vi "Analog Trigger with Interleaving Select.vi"(0 "all channels":cluster{fxp<+/-,12,1>[]}[](array[cluster])=[{[0.0, 0.0, 0.0, 0.0, 0.0, 0.0, 0.0, 0.0, 0.0, 0.0, 0.0, 0.0, 0.0, 0.0, 0.0, 0.0]}, {[0.0, 0.0, 0.0, 0.0, 0.0, 0.0, 0.0, 0.0, 0.0, 0.0, 0.0, 0.0, 0.0, 0.0, 0.0, 0.0]}], 5 "config":T1, 7 "interleaving factor":u16) -> (4 "all channels delayed out":cluster{fxp<+/-,12,1>[]}[](array[cluster]), 6 "triggered":bool)   [LabVIEW 2018, in "GettingStarted_5785_FPGA.lvlib"]
uses:
  GettingStarted_5785_FPGA.lvlib
  1961724d-2c00-4db4-be5f-47e2776cd38e.vi
  db24aacc-3aa9-45e6-b75f-233848c1dcdd.vi
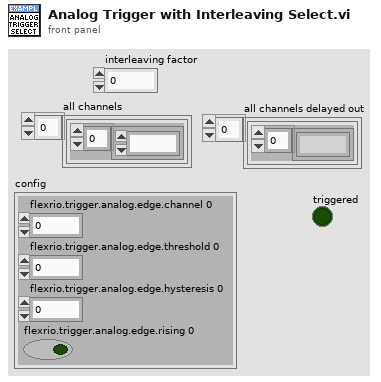
[diagram p1: front panel]
types:
  T1 = cluster{"flexrio.trigger.analog.edge.channel 0":fxp<+,2,2>, "flexrio.trigger.analog.edge.threshold 0":fxp<+/-,32,1>, "flexrio.trigger.analog.edge.hysteresis 0":fxp<+/-,32,1>, "flexrio.trigger.analog.edge.rising 0":bool}
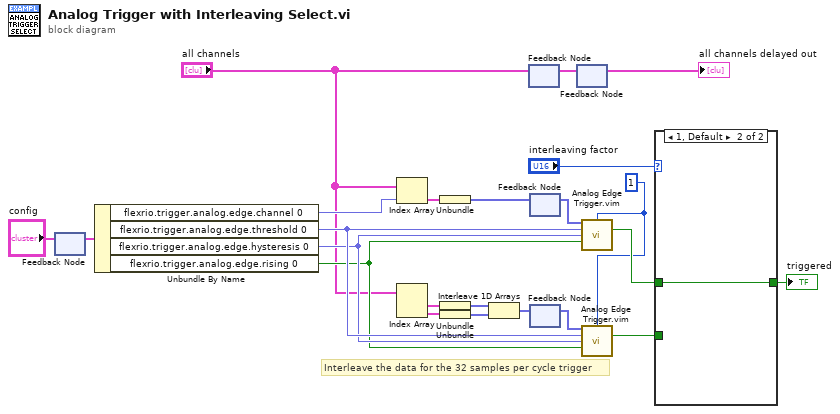
[diagram p0: block diagram]
diagram:
  w10 = u8 1 ("internal pipeline stages")
  # "Interleave the data for the 32 samples per cycle trigger"
  n1 = feedback #1() -> (w8:T1)  [unwired: 1 in]
  n2 = feedback-in #1("config") -> ()
  n3 = Unbundle By Name(w8) -> ("flexrio.trigger.analog.edge.channel 0"=w7:fxp<+,2,2>, "flexrio.trigger.analog.edge.threshold 0"=w6:fxp<+/-,32,1>, "flexrio.trigger.analog.edge.hysteresis 0"=w5:fxp<+/-,32,1>, "flexrio.trigger.analog.edge.rising 0"=w4:bool)
  n4 = Index Array(array="all channels", index=w7) -> (element=w16:cluster{fxp<+/-,12,1>[]})
  n5 = Index Array(array="all channels") -> (element #1=w19:cluster{fxp<+/-,12,1>[]}, element #2=w20:cluster{fxp<+/-,12,1>[]})  [unwired: 2 in]
  n6 = Unbundle(w16) -> (w17:fxp<+/-,12,1>[])
  n7 = Unbundle(w19) -> (w21:fxp<+/-,12,1>[])
  n8 = Unbundle(w20) -> (w22:fxp<+/-,12,1>[])
  n9 = Interleave 1D Arrays(w21, w22) -> (w23:fxp<+/-,12,1>[])
  n10 = feedback #2() -> (w2:cluster{fxp<+/-,12,1>[]}[])  [unwired: 1 in]
  n11 = feedback-in #2("all channels") -> ()
  n12 = feedback #3() -> (w15:fxp<+/-,12,1>[])  [unwired: 1 in]
  n13 = feedback-in #3(w17) -> ()
  n14 = feedback #4() -> (w18:fxp<+/-,12,1>[])  [unwired: 1 in]
  n15 = feedback-in #4(w23) -> ()
  n16 = feedback #5() -> (→"all channels delayed out":cluster{fxp<+/-,12,1>[]}[])  [unwired: 1 in]
  n17 = feedback-in #5(w2) -> ()
  n18 = call "Analog Edge Trigger.vim"("trigger channel data"=w15, "internal pipeline stages"=w10, "requested trigger level"=w6, "requested hysteresis level"=w5, "rising edge"=w4) -> ("triggered"=w12:bool)  [unwired: 7 in, 3 out]
  n19 = call "Analog Edge Trigger.vim"("trigger channel data"=w18, "internal pipeline stages"=w10, "requested trigger level"=w6, "requested hysteresis level"=w5, "rising edge"=w4) -> ("triggered"=w13:bool)  [unwired: 7 in, 3 out]
  n20 = case shown="1, Default" "interleaving factor" {
    tunnel: w13 -> [w24 _]
    tunnel: [w24 w25] -> w11
    tunnel: w12 -> [_ w25]
    frame 2 {
    }
    frame 1, Default {
    }
  }
  "triggered" <- w11
